vi "Read VS input FIFO.vi"(8 "error in (no error)":errorcluster, 10 "CD state in":T1[](array[typedef]), 11 "Refnum in":refnum<k33>) -> (0 "error out (no error)":errorcluster, 2 "CD state out":T1[](array[typedef]))   [LabVIEW 2014, in "UEGO Sim Engine.lvlib"]
uses:
  UEGO Sim Engine.lvlib
  UEGO CD state.ctl
  Shared/UEGO fpga inputs.ctl
  Shared/UEGO fpga outputs.ctl
  Shared/VS input channels.ctl
  Shared/VS output channels.ctl
  Shared/UEGO Sim Shared.lvlib
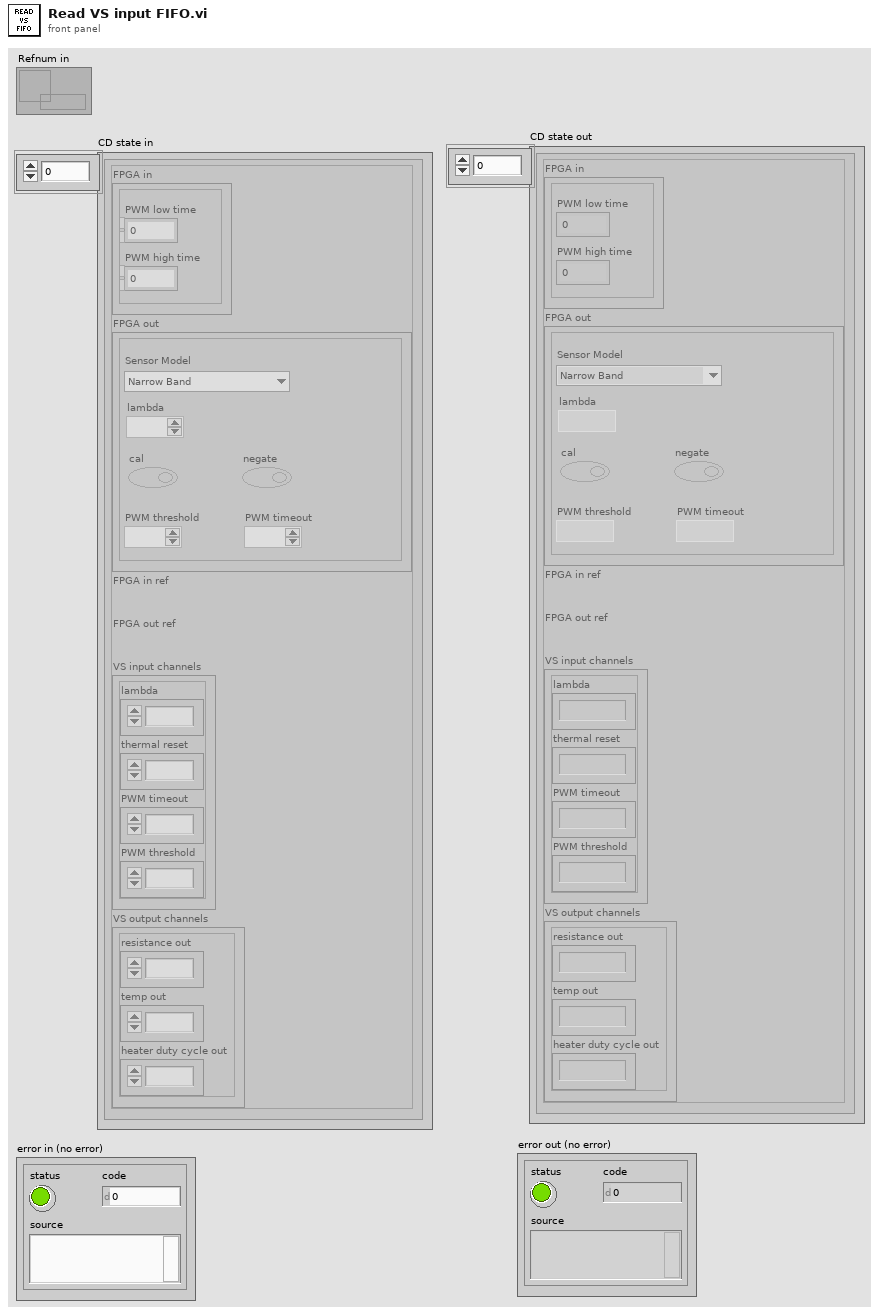
[diagram p1: front panel]
types:
  T1 = typedef "UEGO Sim Engine.lvlib/UEGO CD state.ctl" = cluster{"FPGA in":T2, "FPGA out":T3, "FPGA in ref":refnum<k20>, "FPGA out ref":refnum<k20>, "VS input channels":T5, "VS output channels":T6}
  T2 = typedef "UEGO Sim Shared.lvlib/UEGO fpga inputs.ctl" = cluster{"PWM low time":u32, "PWM high time":u32}
  T3 = typedef "UEGO Sim Shared.lvlib/UEGO fpga outputs.ctl" = cluster{"Sensor Model":T4, "lambda":fxp<+,12,3>, "cal":bool, "negate":bool, "PWM threshold":i16, "PWM timeout":u32}
  T4 = typedef "UEGO Sim Shared.lvlib/sensor models" = enum16{"Narrow Band", "Bosch 4.2", "Bosch 4.9"}
  T5 = typedef "UEGO Sim Shared.lvlib/VS input channels.ctl" = cluster{"lambda":dbl, "thermal reset":dbl, "PWM timeout":dbl, "PWM threshold":dbl}
  T6 = typedef "UEGO Sim Shared.lvlib/VS output channels.ctl" = cluster{"resistance out":dbl, "temp out":dbl, "heater duty cycle out":dbl}
  T7 = cluster{"Array[0]":dbl, "Array[1]":dbl, "Array[2]":dbl, "Array[3]":dbl}
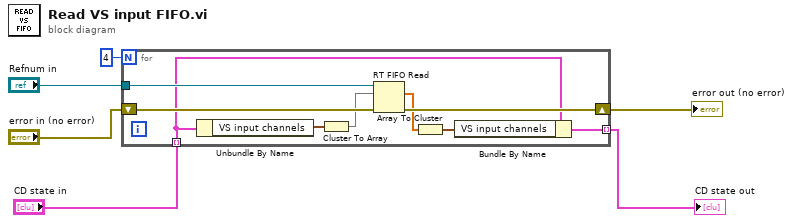
[diagram p0: block diagram]
diagram:
  n1 = for {
    N: 4 -> [_]
    tunnel: "Refnum in" -> [w15]
    shift-right: [w13] -> w3
    shift-left: "error in (no error)" -> [w14]
    tunnel: "CD state in" -> [w10] mode=indexing
    tunnel: [w7] -> w2 mode=indexing
    n2 = Unbundle By Name(w10) -> ("VS input channels"=w12:T5)
    n3 = Cluster To Array(cluster=w12) -> (array=w11:dbl[])
    n4 = RT FIFO Read(0:w15, 1:w11, 3:w14) -> (9:w9:dbl[], 11:w13:errorcluster)  [unwired: 4 out]
    n5 = Array To Cluster(array=w9) -> (cluster=w8:T7)
    n6 = Bundle By Name(cluster=w10, "VS input channels"=w8) -> (w7:T1)
  }
  "error out (no error)" <- w3
  "CD state out" <- w2
